vi "DetectFreezeFinal.vi"(8 "error in (no error)":errorcluster) -> (0 "error out":errorcluster)   [LabVIEW 2013]
doc: "Use this template to build a VI to use as a subVI."
uses:
  DB/DbEnum.ctl
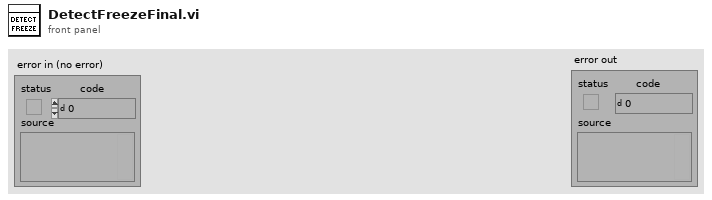
[diagram p1: front panel]
types:
  T1 = typedef "DbEnum.ctl" = enum16{"Write DropletDB", "Init", "Insert Detection Result Data", "Insert Grey Level Result", "Insert Baseline Results", "AddFreezeImagesAtCertainDroplet", "UpdateIncludeDroplet", "Insert Freeze Analysis Results", "GetDropDB", "GetNoFreezedDroplets", "GetGreyLevelAndDiff", "GetGreyLevelatIndexTime", "GetDropletsBoundingBox"}
  T2 = cluster{"ImageIndexArray":u32[], "GreyLevelInBoundingBox":dbl[][], "GLDifference":dbl[][]}
  T3 = typedef "FreezePointData.ctl" = cluster{"Freeze YesNo":cluster{"Freeze Grey Diff value":dbl, "Freeze Point Found":bool, "Freeze Indices":u32[]}[], "Rel Time":u32[]}
  T4 = cluster{"DropletBaseline":dbl[], "DropletBaselineSTD":dbl[]}
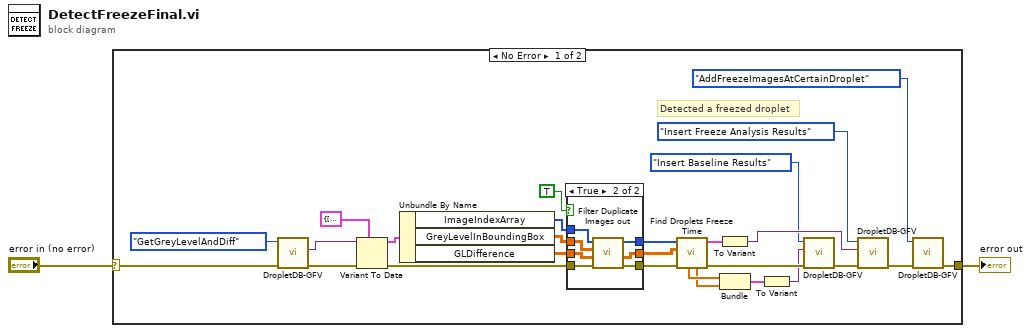
[diagram p0: block diagram]
diagram:
  n1 = case shown="No Error" "error in (no error)" {
    selector: "error in (no error)" -> [w17 w40]
    tunnel: [w16 w40] -> w1
    frame No Error {
      # "Detected a freezed droplet"
      n2 = call "DropletDB-GFV.vi"("error in (no error)"=w17, "Command In"=DbEnum."GetGreyLevelAndDiff") -> ("error out"=w29:errorcluster, "Data out"=w28:variant)  [unwired: 8 in]
      n3 = Variant To Data(error in=w29, type=T2 {"ImageIndexArray"=[], "GreyLevelInBoundingBox"=[], "GLDifference"=[]} ("output cluster"), Variant=w28) -> (data=w26:T2, error out=w24:errorcluster)
      n4 = Unbundle By Name(w26) -> ("ImageIndexArray"=w4:u32[], "GreyLevelInBoundingBox"=w25:dbl[][], "GLDifference"=w3:dbl[][])
      n5 = case shown="True" TRUE {
        tunnel: w4 -> [w32 w39]
        tunnel: w25 -> [_ w38]
        tunnel: w3 -> [w31 w37]
        tunnel: w24 -> [w30 w36]
        tunnel: [w31 w35] -> w5
        tunnel: [w30 w34] -> w23
        tunnel: [w32 w33] -> w6
        frame False {
        }
        frame True {
          n6 = call "Filter Duplicate Images out.vi"("Error In"=w36, "GreyLevel Drops and time Derivative in"=w37, "GreyLevel Drops and time in"=w38, "Rel Time (s) in"=w39) -> ("Error Out"=w34:errorcluster, "GreyLevel Drops and time Derivative out"=w35:dbl[][], "Rel Time (s) out"=w33:u32[])  [unwired: 4 in, 1 out]
        }
      }
      n7 = call "Find Droplets Freeze Time.vi"("Error In"=w23, "GreyLevel Drops and time Derivative in"=w5, "Rel Time Array"=w6) -> ("Error Out"=w22:errorcluster, "FreezeYesNo"=w19:T3, "DropletBaselineSTD"=w20:dbl[], "DropletBaseline"=w21:dbl[])  [unwired: 5 in]
      n8 = To Variant(anything=w19) -> (Variant=w14:variant)
      n9 = Bundle("DropletBaseline"=w21, "DropletBaselineSTD"=w20) -> (w9:T4)  [unwired: 1 in]
      n10 = To Variant(anything=w9) -> (Variant=w8:variant)
      n11 = call "DropletDB-GFV.vi"("error in (no error)"=w22, "Data in"=w8, "Command In"=DbEnum."Insert Baseline Results") -> ("error out"=w7:errorcluster)  [unwired: 7 in, 1 out]
      n12 = call "DropletDB-GFV.vi"("error in (no error)"=w7, "Data in"=w14, "Command In"=DbEnum."Insert Freeze Analysis Results") -> ("error out"=w11:errorcluster)  [unwired: 7 in, 1 out]
      n13 = call "DropletDB-GFV.vi"("error in (no error)"=w11, "Command In"=DbEnum."AddFreezeImagesAtCertainDroplet") -> ("error out"=w16:errorcluster)  [unwired: 8 in, 1 out]
    }
    frame Error {
    }
  }
  "error out" <- w1
